vi "Escape.vi"(6 "Reset cursor (T)":bool=TRUE, 8 "error in":errorcluster, 11 "Data in":T1={"Class"={"Ants"=refnum, "Layer"=refnum, "Templates"=refnum, "Icon"=refnum, "Glyph"=refnum, "Settings"=refnum, "Tools"=refnum}, "Ref"={"Add Layer"=refnum, "Remove Layer"=refnum, "Line Text"=[], "Body Text Spec"=refnum, "DNL_Font"=refnum, "glyph path str"=refnum, "templates path str"=refnum, "Arrow Up"=refnum, "Arrow Down"=refnum, "IE VI Ref"=refnum, "Glyphs tree"=refnum, "Templates tree"=refnum, "Layer Icon Text"=refnum, "Layer Template"=refnum, "Body Text"=refnum, "Search Templates"=refnum, "TextMarker"=refnum, "Tab Control"=refnum, "Search Glyphs"=refnum, "Line Color"=refnum, "DNL_Glyphs []"=refnum, "Fill Color"=refnum, "Tools"=refnum, "Icon"=refnum, "Preview"=refnum, "Ants"=refnum, "Terminals"=refnum, "menu reference"=refnum, "LayerNames"=[], "GlyphLoadAnimation"=refnum, "TemplateLoadAnimation"=refnum, "refreshGlyphs"=refnum, "refreshTemplates"=refnum}, "Support"={"AntsRect"={"left"=0, "top"=0, "right"=0, "bottom"=0}, "Mouse Move Coords"={"Horizontal"=0, "Vertical"=0}, "Mouse Down Coords"={"Horizontal"=0, "Vertical"=0}, "Temp Coord"={"Horizontal"=0, "Vertical"=0}, "Action"=enum."Default", "Edge Color"=4914962, "Fill Color"=16860, "Mouse Down?"=FALSE, "Draft Mode?"=FALSE, "Temp Icon"=bytes[3102], "CTRL Pressed"=FALSE, "Move Selection?"=FALSE, "AntsRect Orig"={"left"=0, "top"=0, "right"=0, "bottom"=0}, "Text"="", "TM Set?"=FALSE, "Mouse inside icon?"=FALSE, "Tool (old value)"=0, "Pencil Move Color"=0, "Swap Colors?"=FALSE, "Shift pressed?"=FALSE}}) -> (0 "error out":errorcluster, 3 "Data out":T1={"Class"={"Ants"=refnum, "Layer"=refnum, "Templates"=refnum, "Icon"=refnum, "Glyph"=refnum, "Settings"=refnum, "Tools"=refnum}, "Ref"={"Add Layer"=refnum, "Remove Layer"=refnum, "Line Text"=[], "Body Text Spec"=refnum, "DNL_Font"=refnum, "glyph path str"=refnum, "templates path str"=refnum, "Arrow Up"=refnum, "Arrow Down"=refnum, "IE VI Ref"=refnum, "Glyphs tree"=refnum, "Templates tree"=refnum, "Layer Icon Text"=refnum, "Layer Template"=refnum, "Body Text"=refnum, "Search Templates"=refnum, "TextMarker"=refnum, "Tab Control"=refnum, "Search Glyphs"=refnum, "Line Color"=refnum, "DNL_Glyphs []"=refnum, "Fill Color"=refnum, "Tools"=refnum, "Icon"=refnum, "Preview"=refnum, "Ants"=refnum, "Terminals"=refnum, "menu reference"=refnum, "LayerNames"=[], "GlyphLoadAnimation"=refnum, "TemplateLoadAnimation"=refnum, "refreshGlyphs"=refnum, "refreshTemplates"=refnum}, "Support"={"AntsRect"={"left"=0, "top"=0, "right"=0, "bottom"=0}, "Mouse Move Coords"={"Horizontal"=0, "Vertical"=0}, "Mouse Down Coords"={"Horizontal"=0, "Vertical"=0}, "Temp Coord"={"Horizontal"=0, "Vertical"=0}, "Action"=enum."Default", "Edge Color"=4914962, "Fill Color"=16860, "Mouse Down?"=FALSE, "Draft Mode?"=FALSE, "Temp Icon"=bytes[3102], "CTRL Pressed"=FALSE, "Move Selection?"=FALSE, "AntsRect Orig"={"left"=0, "top"=0, "right"=0, "bottom"=0}, "Text"="", "TM Set?"=FALSE, "Mouse inside icon?"=FALSE, "Tool (old value)"=0, "Pencil Move Color"=0, "Swap Colors?"=FALSE, "Shift pressed?"=FALSE}})   [LabVIEW 2020]
uses:
  Class/Ants/Ants.lvclass
  Class/FakedArray/FakedArray.lvclass
  vi.lib/LabVIEW Icon API/lv_icon/Classes/Icon/Icon.lvclass
  Class/Icon Library/Glyph.lvclass
  Class/Settings/Settings.lvclass
  Class/Tools/Tools Paint.lvclass
  Controls/SupportClass_Action.ctl
  <vilib>/Utility/miscctls.llb/LVPoint32TypeDef.ctl
  vi.lib/LabVIEW Icon API/lv_icon/Controls/IEColor.ctl
  Controls/SupportClass.ctl
  Controls/References Cluster.ctl
  vi.lib/LabVIEW Icon API/lv_icon/lv_icon.lvlib
  Controls/IE Classes.ctl
  Controls/Global Data.ctl
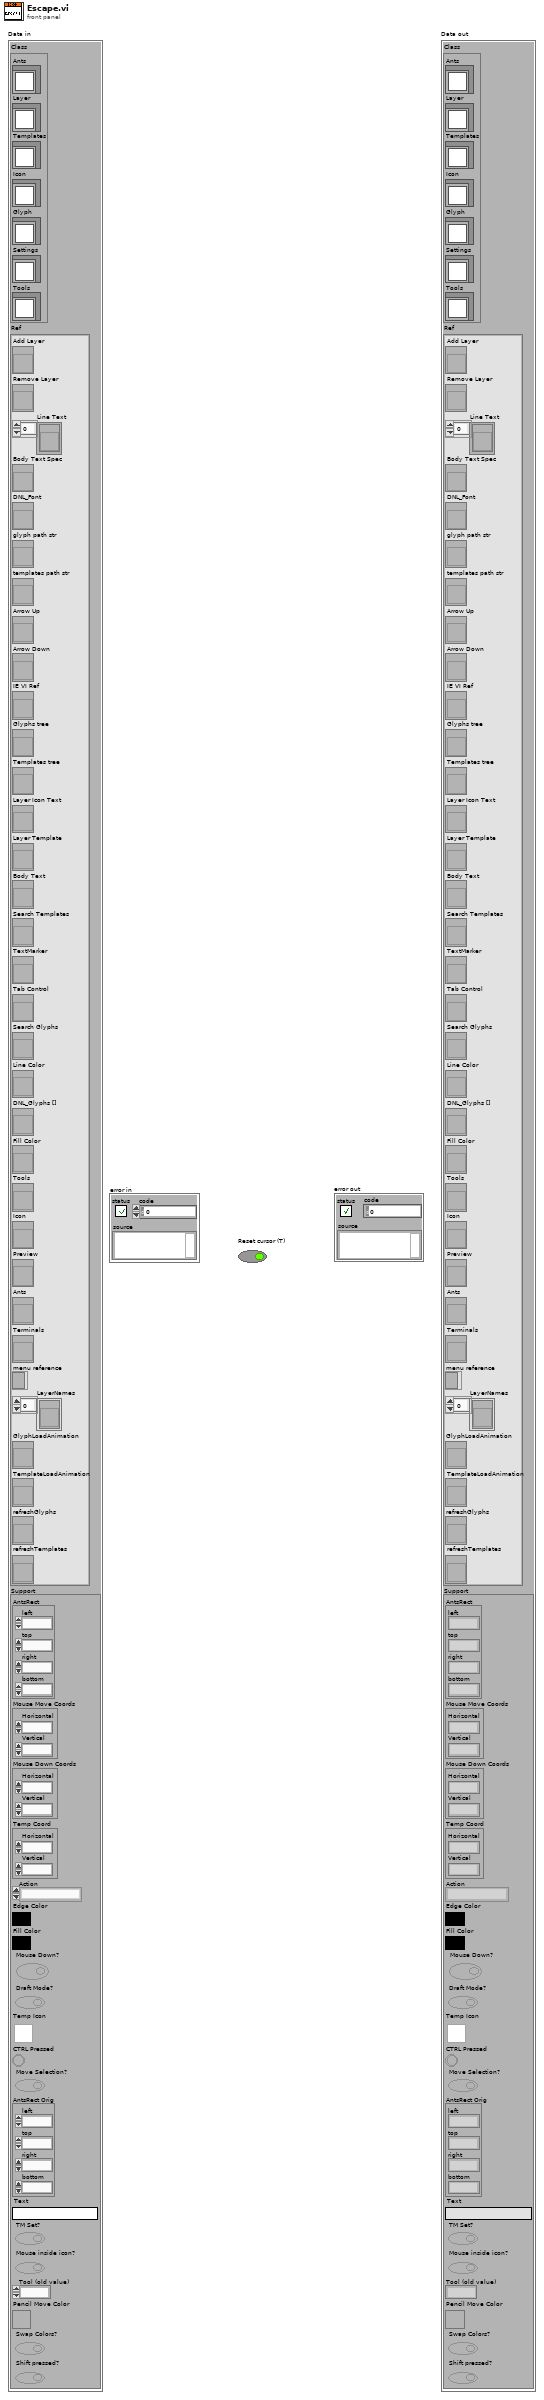
[diagram p1: front panel]
types:
  T1 = typedef "lv_icon.lvlib/Global Data.ctl" = cluster{"Class":T2, "Ref":T3, "Support":T4}
  T2 = typedef "IE Classes.ctl" = cluster{"Ants":refnum<class "Ants.lvclass">, "Layer":refnum<class "FakedArray.lvclass">, "Templates":refnum<class "FakedArray.lvclass">, "Icon":refnum<class "Icon.lvclass">, "Glyph":refnum<class "Glyph.lvclass">, "Settings":refnum<class "Settings.lvclass">, "Tools":refnum<class "Tools Paint.lvclass">}
  T3 = typedef "lv_icon.lvlib/References Cluster.ctl" = cluster{"Add Layer":refnum<vi>, "Remove Layer":refnum<vi>, "Line Text":refnum<vi>[], "Body Text Spec":refnum<vi>, "DNL_Font":refnum<vi>, "glyph path str":refnum<vi>, "templates path str":refnum<vi>, "Arrow Up":refnum<vi>, "Arrow Down":refnum<vi>, "IE VI Ref":refnum<vi>, "Glyphs tree":refnum<vi>, "Templates tree":refnum<vi>, "Layer Icon Text":refnum<vi>, "Layer Template":refnum<vi>, "Body Text":refnum<vi>, "Search Templates":refnum<vi>, "TextMarker":refnum<vi>, "Tab Control":refnum<vi>, "Search Glyphs":refnum<vi>, "Line Color":refnum<vi>, "DNL_Glyphs []":refnum<vi>, "Fill Color":refnum<vi>, "Tools":refnum<vi>, "Icon":refnum<vi>, "Preview":refnum<vi>, "Ants":refnum<vi>, "Terminals":refnum<vi>, "menu reference":refnum<k9>, "LayerNames":refnum<vi>[], "GlyphLoadAnimation":refnum<vi>, "TemplateLoadAnimation":refnum<vi>, "refreshGlyphs":refnum<vi>, "refreshTemplates":refnum<vi>}
  T4 = typedef "SupportClass.ctl" = cluster{"AntsRect":cluster{"left":i16, "top":i16, "right":i16, "bottom":i16}, "Mouse Move Coords":T5, "Mouse Down Coords":T5, "Temp Coord":T5, "Action":T6, "Edge Color":T7, "Fill Color":T7, "Mouse Down?":bool, "Draft Mode?":bool, "Temp Icon":picture, "CTRL Pressed":bool, "Move Selection?":bool, "AntsRect Orig":cluster{"left":i16, "top":i16, "right":i16, "bottom":i16}, "Text":string, "TM Set?":bool, "Mouse inside icon?":bool, "Tool (old value)":u32, "Pencil Move Color":u32, "Swap Colors?":bool, "Shift pressed?":bool}
  T5 = typedef "LVPoint32TypeDef.ctl" = cluster{"Horizontal":i32, "Vertical":i32}
  T6 = typedef "SupportClass_Action.ctl" = enum16{"Default", "Move Selection", "Glyph Library", "Tool"}
  T7 = typedef "IEColor.ctl" = u32
  T8 = cluster{"Horizontal":i32, "Vertical":i32, "Vertical 2":i32, "Vertical 3":i32}
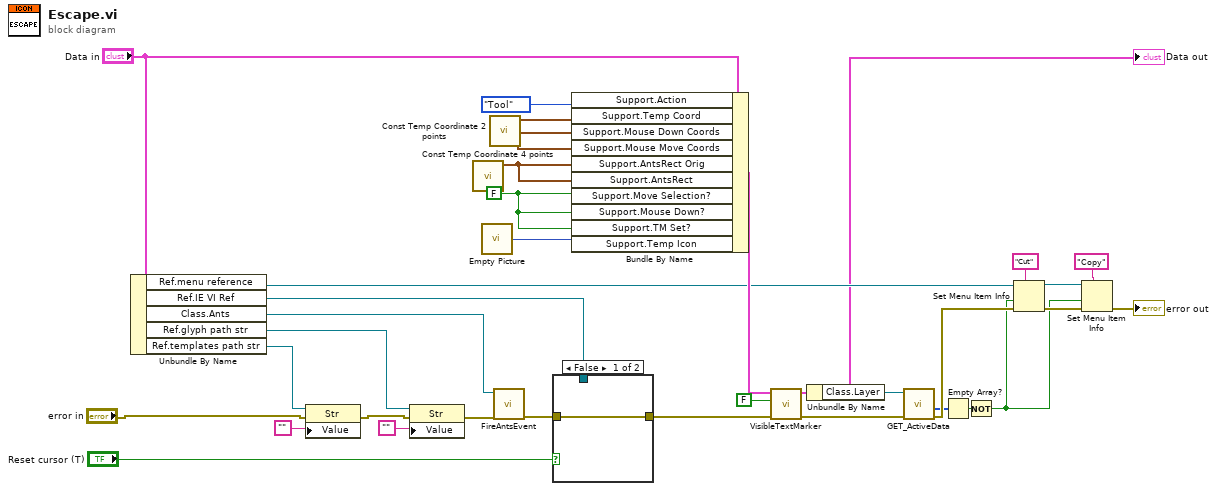
[diagram p0: block diagram]
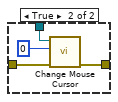
[diagram p2: hidden frame]
diagram:
  w27 = FALSE ("Mouse Down?")
  n1 = Unbundle By Name("Data in") -> ("Ref.menu reference"=w20:refnum<k9>, "Ref.IE VI Ref"=w24:refnum<vi>, "Class.Ants"=w25:refnum<class "Ants.lvclass">, "Ref.glyph path str"=w6:refnum<vi>, "Ref.templates path str"=w2:refnum<vi>)
  n2 = property class="Str"(reference=w2, error in="error in", "Value"="") -> (error out=w3:errorcluster)  [unwired: 1 out]
  n3 = property class="Str"(reference=w6, error in=w3, "Value"="") -> (error out=w7:errorcluster)  [unwired: 1 out]
  n4 = call "Const Temp Coordinate 4 points.vi"() -> ("Const Temp Coordinate"=w33:T8)  [unwired: 11 out]
  n5 = call "Empty Picture"() -> ("empty picture"=w30:picture)
  n6 = call "Const Temp Coordinate 2 points.vi"() -> ("Const Temp Coordinate"=w31:T5)  [unwired: 11 out]
  n7 = call "FireAntsEvent.vi"("error in (no error)"=w7, "Ants in"=w25) -> ("error out"=w29:errorcluster)  [unwired: 2 in, 7 out]
  n8 = case shown="False" "Reset cursor (T)" {
    tunnel: w29 -> [w34 w38]
    tunnel: [w34 w37] -> w28
    tunnel: w24 -> [_ w35]
    frame False {
    }
    frame True {
      n9 = call "Change Mouse Cursor.vi"("error in (no error)"=w38, "icon"=u16 0, "VI reference (current VI)"=w35) -> ("error out"=w37:errorcluster)  [unwired: 8 out]
    }
  }
  n10 = Bundle By Name(cluster="Data in", "Support.Action"=SupportClass_Action."Tool" ("Action"), "Support.Temp Coord"=w31, "Support.Mouse Down Coords"=w31, "Support.Mouse Move Coords"=w31, "Support.AntsRect Orig"=w33, "Support.AntsRect"=w33, "Support.Move Selection?"=w27, "Support.Mouse Down?"=w27, "Support.TM Set?"=w27, "Support.Temp Icon"=w30) -> (w23:T1)
  n11 = call "VisibleTextMarker.vi"("error in (no error)"=w28, "Visible"=FALSE, "Data in"=w23) -> ("error out"=w13:errorcluster, "Data out"=w14:T1)  [unwired: 1 in, 6 out]
  "Data out" <- w14
  n12 = Unbundle By Name(w14) -> ("Class.Layer"=w12:refnum<class "FakedArray.lvclass">)
  n13 = call-dynamic "GET_ActiveData.vi"("error in (no error)"=w13, "FakedArray in"=w12) -> ("error out"=w11:errorcluster, "Active Data []"=w10:i32[])  [unwired: 4 in, 4 out]
  n14 = Empty Array?(array=w10) -> (empty?=w9:bool)
  n15 = Not(x=w9) -> (.not. x?=w8:bool)
  n16 = Set Menu Item Info(7:"Cut" ("item tag"), 8:w11, 9:w8, 11:w20) -> (0:w18:errorcluster, 3:w16:refnum<k9>)  [unwired: 3 out]
  n17 = Set Menu Item Info(7:"Copy" ("item tag"), 8:w18, 9:w8, 11:w16) -> (0:→"error out":errorcluster)  [unwired: 4 out]
